vi "CRYGet Current CurLib Listbox.vi"() -> (0 "bResult":bool, 2 "CurLib Tree":refnum<vi>, 3 "Type":enum16{"Curves", "Values", "Results", "WFM"}(ring))   [LabVIEW 2013]
uses:
  Global/CRYCurve Library Global.vi
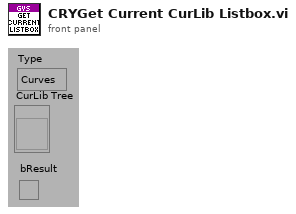
[diagram p1: front panel]
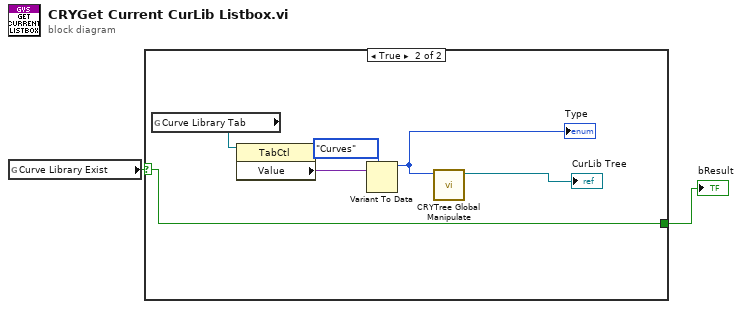
[diagram p0: block diagram]
diagram:
  n1 = global read "CRYCurve Library Global.vi" "Curve Library Exist"() -> (w2:bool)
  n2 = case shown="True" w2 {
    selector: w2 -> [w3 w6]
    tunnel: [w3 w6] -> w1
    frame False {
    }
    frame True {
      n3 = global read "CRYCurve Library Global.vi" "Curve Library Tab"() -> (w9:refnum<vi>)
      n4 = property on="Property Node" class="TabCtl"(reference=w9) -> ("Value"=w7:variant)  [unwired: 1 in, 2 out]
      n5 = Variant To Data(type=enum32{"Curves", "Values", "Results", "WFM"}."Curves" ("Type"), Variant=w7) -> (data=w4:enum32{"Curves", "Values", "Results", "WFM"})  [unwired: 1 in, 1 out]
      "Type" <- w4
      n6 = call "CRYTree Global Manipulate.vi"("Type In"=w4) -> ("Tree/Curve Tree"=→"CurLib Tree":refnum<vi>)  [unwired: 7 in, 3 out]
    }
  }
  "bResult" <- w1
